vi "calculate_derived_values.vi"(11 "scan specification":T2) -> (3 "derived values":T1)   [LabVIEW 2010]
uses:
  scan_specification_cluster.ctl
  derived_values_cluster.ctl
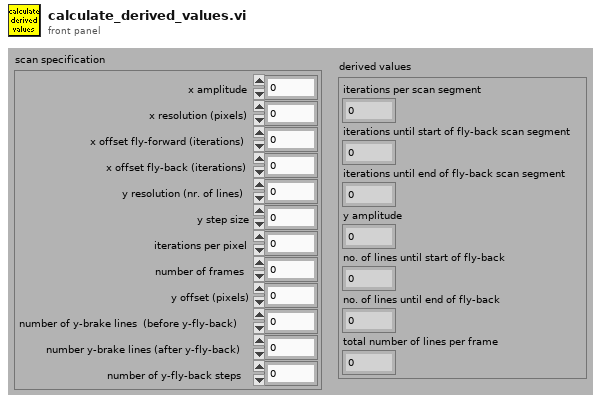
[diagram p1: front panel]
types:
  T1 = typedef "derived_values_cluster.ctl" = cluster{"iterations per scan segment":u16, "iterations until start of fly-back scan segment":u16, "iterations until end of fly-back scan segment":u16, "y amplitude":u16, "no. of lines until start of fly-back":u16, "no. of lines until end of fly-back":u16, "total number of lines per frame ":u16}
  T2 = typedef "scan_specification_cluster.ctl" = cluster{"x amplitude":u16, "x resolution (pixels)":u16, "x offset fly-forward (iterations)":u16, "x offset fly-back (iterations)":u16, "y resolution (nr. of lines)":u16, "y step size":u16, "iterations per pixel":u16, "number of frames":i32, "y offset (pixels)":u16, "number of y-brake lines  (before y-fly-back)":u16, "number y-brake lines (after y-fly-back)":u16, "number of y-fly-back steps":u16}
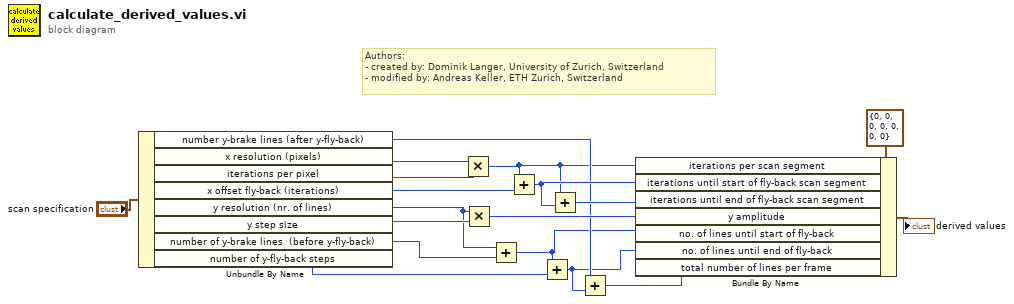
[diagram p0: block diagram]
diagram:
  # "Authors: \n- created by: Dominik Langer, University of Zurich, Switzerland\n- modified by: Andreas Keller, ETH Zurich, Switzerland"
  n1 = Unbundle By Name("scan specification") -> ("number y-brake lines (after y-fly-back)"=w6:u16, "x resolution (pixels)"=w15:u16, "iterations per pixel"=w14:u16, "x offset fly-back (iterations)"=w13:u16, "y resolution (nr. of lines)"=w8:u16, "y step size"=w10:u16, "number of y-brake lines  (before y-fly-back)"=w7:u16, "number of y-fly-back steps"=w3:u16)
  n2 = Multiply(x=w15, y=w14) -> (x*y=w2:u16)
  n3 = Multiply(x=w8, y=w10) -> (x*y=w9:u16)
  n4 = Add(x=w8, y=w7) -> (x+y=w4:u16)
  n5 = Add(x=w2, y=w13) -> (x+y=w12:u16)
  n6 = Add(x=w4, y=w3) -> (x+y=w5:u16)
  n7 = Add(x=w2, y=w12) -> (x+y=w11:u16)
  n8 = Add(x=w6, y=w5) -> (x+y=w1:u16)
  n9 = Bundle By Name(cluster=T1 {"iterations per scan segment"=0, "iterations until start of fly-back scan segment"=0, "iterations until end of fly-back scan segment"=0, "y amplitude"=0, "no. of lines until start of fly-back"=0, "no. of lines until end of fly-back"=0, "total number of lines per frame "=0} ("derived values"), "iterations per scan segment"=w2, "iterations until start of fly-back scan segment"=w12, "iterations until end of fly-back scan segment"=w11, "y amplitude"=w9, "no. of lines until start of fly-back"=w4, "no. of lines until end of fly-back"=w5, "total number of lines per frame"=w1) -> (→"derived values":T1)
